vi "UHR-Fleezers Control (host) - 12.6.vi"() -> ()   [LabVIEW 2012] (continued)
      event "Move Cap. 2 (ADig Top)": Value Change {
        n240 = event-data() -> ()  [unwired: 1 in, 5 out]
        n241 = local write "Move Cap. 2 (ADig Top)"(FALSE ("Move Cap. 2 (ADig Left)")) -> ()
        n242 = flat-sequence {
          tunnel: w445 -> [w448]
          tunnel: w446 -> [w449]
          tunnel: [w449] -> w443
          tunnel: [w448] -> w442
          tunnel: w443 -> [w452]
          tunnel: w442 -> [w451]
          frame #0 {
            n243 = property on="Sample Channel\nFlow" class="Bool (strict)"("Val(Sgnl)"="Cap 2 Samp Flow ON") -> ()  [unwired: 2 in, 2 out]
          }
          frame #1 {
            w450 = FALSE ("Value (Signaling)")
            n244 = local read "Saved Stage Positions"() -> (w462:dbl[][])
            n245 = local write "Stage Moving"(TRUE ("Stage Moving")) -> ()
            n246 = Array Subset(array=w462, index (row)=1 ("index"), length (row)=1 ("length"), index (col)=1 ("index"), length (col)=3 ("length")) -> (w459:dbl[][])
            n247 = Reshape Array(w459, 3 ("dimension size")) -> (w457:dbl[])
            n248 = property on="Trap 1 (ON/OFF)" class="Bool (strict)"("Val(Sgnl)"=w450) -> ()  [unwired: 2 in, 2 out]
            n249 = property on="Trap 1 (ON/OFF)" class="Bool (strict)"("Val(Sgnl)"=w450) -> ()  [unwired: 2 in, 2 out]
            n250 = Array To Cluster(array=w457) -> (cluster=w456:cluster{"[0]":dbl, "[1]":dbl, "[2]":dbl})
            n251 = call "Set Stage Position.vi"("Position"=w456, "error in"=w451, "VISA resource name in"=w452) -> ("error out"=w455:errorcluster)  [unwired: 2 out]
            n252 = local write "Stage Control Serial Error"(w455) -> ()
          }
          frame #2 {
            n253 = local write "Stage Moving"(FALSE ("Stage Moving")) -> ()
            n254 = call <vilib>:"Beep.vi"() -> ()  [unwired: 3 in, 9 out]
            n255 = case shown="True" "Cap 2 Flow ON" {
              frame False {
              }
              frame True {
                n256 = property on="Inject Pump 3" class="Bool (strict)"("Val(Sgnl)"=TRUE ("Value (Signaling)")) -> ()  [unwired: 2 in, 2 out]
              }
            }
          }
          frame #3 {
            n257 = property on="Sample Channel\nFlow" class="Bool (strict)"("Val(Sgnl)"=FALSE ("Value (Signaling)")) -> ()  [unwired: 2 in, 2 out]
            n258 = case shown="False" "Cap. 2 BD T1?\n(ADig T1, DNA T2)" {
              tunnel: "Cap 2 T ON" -> [w471 w472]
              frame False {
                n259 = property on="Trap 2 (ON/OFF)" class="Bool (strict)"("Val(Sgnl)"=w471) -> ()  [unwired: 2 in, 2 out]
              }
              frame True {
                n260 = property on="Trap 1 (ON/OFF)" class="Bool (strict)"("Val(Sgnl)"=w472) -> ()  [unwired: 2 in, 2 out]
              }
            }
            n261 = property on="Got ADig bead" class="Bool"("Key Focus"=TRUE) -> ()  [unwired: 2 in, 2 out]
          }
        }
      }
      event "Initialize Blue Laser": Value Change {
        n262 = event-data() -> ()  [unwired: 1 in, 5 out]
        n263 = flat-sequence {
          tunnel: w473 -> [w492]
          frame #0 {
            n264 = Concatenate Strings("slmp ", "Blue Laser\nModulation\nPower (mW)") -> (w491:string)
            n265 = call "serial write macro.vi"("String"=w491, "Delay (ms)"="Delay (ms)", "VISA resource name"=w492) -> ("read buffer"=w480:string, "error out"=w481:errorcluster, "VISA resource name out"=w488:refnum<visa-resource-name>)
            n266 = local write "read blue buffer"(w480) -> ()
            n267 = local write "Blue Error Out"(w481) -> ()
            n268 = call "serial write macro.vi"("String"="sdmes 1", "Delay (ms)"="Delay (ms)", "VISA resource name"=w488) -> ("read buffer"=w478:string, "error out"=w479:errorcluster, "VISA resource name out"=w486:refnum<visa-resource-name>)
            n269 = local write "Blue Error Out"(w479) -> ()
            n270 = local write "read blue buffer"(w478) -> ()
            n271 = call "serial write macro.vi"("String"="sames 1", "Delay (ms)"="Delay (ms)", "VISA resource name"=w486) -> ("read buffer"=w475:string, "error out"=w477:errorcluster, "VISA resource name out"=w483:refnum<visa-resource-name>)
            n272 = local write "read blue buffer"(w475) -> ()
            n273 = local write "Blue Error Out"(w477) -> ()
            n274 = call "serial write macro.vi"("String"="l1", "Delay (ms)"="Delay (ms)", "VISA resource name"=w483) -> ("read buffer"=w474:string, "error out"=w476:errorcluster)  [unwired: 1 out]
            n275 = local write "read blue buffer"(w474) -> ()
            n276 = local write "Blue Error Out"(w476) -> ()
          }
          frame #1 {
            n277 = local write "Initialize Blue Laser"(FALSE ("Initialize")) -> ()
          }
        }
      }
      event "Blue Laser Modluation Mode": Value Change {
        # "Changes the type of modulation for the blue laser"
        n278 = event-data() -> ()  [unwired: 1 in, 5 out]
        n279 = case shown="\"Constant Power\"" "Blue Laser Modluation Mode" {
          tunnel: ["sdmes 1" w510 "sdmes 1" "sdmes 0"] -> w495
          tunnel: ["sames 1" "cp" "sames 0" "sames 1"] -> w494
          frame "Digital + Analog", Default {
          }
          frame "Constant Power" {
            n280 = local read "Blue Laser\nModulation\nPower (mW)"() -> (w513:string)
            n281 = Decimal String To Number(string=w513) -> (number=w509:i32)  [unwired: 2 in, 1 out]
            n282 = Divide(x=w509, y=1000) -> (x/y=w507:dbl)
            n283 = Number To Fractional String(number=w507) -> (F-format string=w508:string)  [unwired: 3 in]
            n284 = Concatenate Strings("p ", w508) -> (w510:string)
          }
          frame "Digital Only" {
          }
          frame "Analog Only" {
          }
        }
        n285 = local read "Delay (ms)"() -> (w504:i32)
        n286 = call "serial write macro.vi"("String"=w495, "Delay (ms)"=w504, "VISA resource name"=w501) -> ("read buffer"=w502:string, "error out"=w503:errorcluster, "VISA resource name out"=w496:refnum<visa-resource-name>)
        n287 = local write "read blue buffer"(w502) -> ()
        n288 = local write "Blue Error Out"(w503) -> ()
        n289 = local read "Delay (ms)"() -> (w499:i32)
        n290 = call "serial write macro.vi"("String"=w494, "Delay (ms)"=w499, "VISA resource name"=w496) -> ("read buffer"=w497:string, "error out"=w498:errorcluster)  [unwired: 1 out]
        n291 = local write "Blue Error Out"(w498) -> ()
        n292 = local write "read blue buffer"(w497) -> ()
      }
      event "Blue Laser\nModulation\nPower (mW)": Value Change {
        n293 = event-data() -> ()  [unwired: 1 in, 5 out]
        n294 = local read "Blue Laser\nModulation\nPower (mW)"() -> (w520:string)
        n295 = local read "Blue Laser Modluation Mode"() -> (w521:string)
        n296 = case shown="\"Constant Power\"" w521 {
          tunnel: w520 -> [w527 w534]
          tunnel: [w526 w533] -> w519
          frame "Constant Power" {
            # "Different command to change constant power instead of modulation power"
            n297 = Decimal String To Number(string=w527) -> (offset past number=w532:i32)  [unwired: 2 in, 1 out]
            n298 = Divide(x=w532, y=1000) -> (x/y=w530:dbl)
            n299 = Number To Fractional String(number=w530) -> (F-format string=w528:string)  [unwired: 3 in]
            n300 = Concatenate Strings("p ", w528) -> (w526:string)
          }
          frame Default {
            n301 = Concatenate Strings("slmp ", w534) -> (w533:string)
          }
        }
        n302 = local read "Delay (ms)"() -> (w524:i32)
        n303 = call "serial write macro.vi"("String"=w519, "Delay (ms)"=w524, "VISA resource name"=w525) -> ("read buffer"=w523:string, "error out"=w522:errorcluster)  [unwired: 1 out]
        n304 = local write "Blue Error Out"(w522) -> ()
        n305 = local write "read blue buffer"(w523) -> ()
      }
      event "Send string\nto Blue Laser": Value Change {
        n306 = event-data() -> ()  [unwired: 1 in, 5 out]
        n307 = flat-sequence {
          tunnel: w536 -> [w541]
          frame #0 {
            n308 = local read "Delay (ms)"() -> (w538:i32)
            n309 = call "serial write macro.vi"("String"="command string", "Delay (ms)"=w538, "VISA resource name"=w541) -> ("read buffer"=w539:string, "error out"=→"Blue Error Out":errorcluster)  [unwired: 1 out]
            "read blue buffer" <- w539
            n310 = String Length(string=w539) -> (length=→"length":i32)
            "command string sent" <- "command string"
          }
          frame #1 {
            n311 = local write "Send string\nto Blue Laser"(FALSE ("Send string")) -> ()
          }
        }
      }
      event "Read Harvard": Value Change {
        n312 = event-data() -> ()  [unwired: 1 in, 5 out]
        n313 = Concatenate Strings("write buffer", "\r") -> (w548:string)
        n314 = VISA Write(VISA resource name=w546, write buffer=w548, error in (no error)=w545) -> (VISA resource name out=w557:refnum<visa-resource-name>, error out=w556:errorcluster)  [unwired: 1 out]
        n315 = stacked-sequence {
          tunnel: [w560] -> w555
          tunnel: w557 -> [w560]
          tunnel: w556 -> [w559]
          tunnel: [w559] -> w550
          frame #0 {
            n316 = Wait (ms)(milliseconds to wait=50) -> ()  [unwired: 1 out]
          }
        }
        n317 = property class="Instr"(reference=w555, error in=w550) -> (reference out=w554:refnum<visa-resource-name>, error out=w552:errorcluster, "Serial Settings:Number of Bytes at Serial Port"=w553:u32)
        "Serial Settings:Number of Bytes at Serial Port" <- w553
        n318 = VISA Read(VISA resource name=w554, byte count=w553, error in (no error)=w552) -> (read buffer=w551:string)  [unwired: 3 out]
        "read buffer" <- w551
        n319 = Fract/Exp String To Number(string=w551) -> ()  [unwired: 5 out]
      }
      event "+z", "-z": Value Change {
        n320 = event-data() -> ()  [unwired: 1 in, 5 out]
        n321 = flat-sequence {
          tunnel: w561 -> [w583]
          tunnel: w562 -> [w563]
          frame #0 {
            n322 = call "Read Stage Position.vi"("error in"=w583, "VISA resource name in"=w563) -> ("Current Position"=w568:cluster{dbl, dbl, dbl}, "error out"=w581:errorcluster, "VISA resource name out"=w582:refnum<visa-resource-name>)  [unwired: 1 out]
            n323 = local read "Saved Stage Positions"() -> (w592:dbl[][])
            n324 = Divide(x="z nudge increment (um)", y=1000.0) -> (x/y=w580:dbl)
            n325 = Boolean To (0,1)(Boolean="+z") -> (0, 1=w572:i16)
            n326 = Boolean To (0,1)(Boolean="-z") -> (0, 1=w573:i16)
            n327 = Array Subset(array=w592, index (row)=1 ("index"), length (row)=1 ("length"), index (col)=1 ("index"), length (col)=3 ("length")) -> (w589:dbl[][])
            n328 = Multiply(x=w572, y=w580) -> (x*y=w576:dbl)
            n329 = Multiply(x=w573, y=w580) -> (x*y=w574:dbl)
            n330 = Unbundle(w568) -> (w566:dbl, w565:dbl, w569:dbl)
            n331 = Negate(x=w574) -> (-x=w575:dbl)
            n332 = Reshape Array(w589, 3 ("dimension size")) -> (w587:dbl[])
            n333 = Add(x=w576, y=w575) -> (x+y=w577:dbl)
            n334 = Array To Cluster(array=w587) -> ()  [unwired: 1 out]
            n335 = Add(x=w577, y=w569) -> (x+y=w567:dbl)
            n336 = Bundle(cluster=w568, w566, w565, w567) -> (w564:cluster{dbl, dbl, dbl})
            n337 = call "Set Stage Position.vi"("Position"=w564, "error in"=w581, "VISA resource name in"=w582) -> ("error out"=w586:errorcluster)  [unwired: 2 out]
            n338 = local write "Stage Moving"(TRUE ("Stage Moving")) -> ()
            n339 = local write "Stage Control Serial Error"(w586) -> ()
          }
          frame #1 {
            n340 = local write "Stage Moving"(FALSE ("Stage Moving")) -> ()
            n341 = call <vilib>:"Beep.vi"() -> ()  [unwired: 3 in, 9 out]
          }
        }
      }
      event "Cal/Data Acq. Spot": Value Change {
        n342 = event-data() -> ()  [unwired: 1 in, 5 out]
        n343 = flat-sequence {
          tunnel: w601 -> [w605]
          tunnel: w602 -> [w606]
          tunnel: [w606] -> w598
          tunnel: [w605] -> w597
          tunnel: w598 -> [w611]
          tunnel: w597 -> [w610]
          tunnel: ["Cal @ (MHz)"] -> w595
          tunnel: [w615] -> w599
          tunnel: w595 -> [w615]
          tunnel: w599 -> [w624]
          tunnel: ["W/ Offset 1"] -> w596
          tunnel: w599 -> [w645]
          tunnel: w596 -> [w643]
          frame #0 {
            n344 = property on="Sample Channel\nFlow" class="Bool (strict)"("Val(Sgnl)"="Daq spot flow on") -> ()  [unwired: 2 in, 2 out]
            n345 = Wait (ms)(milliseconds to wait=u32 250) -> ()  [unwired: 1 out]
          }
          frame #1 {
            n346 = local read "Saved Stage Positions"() -> (w608:dbl[][])
            n347 = property on="Trap Delta (MHz)" class="DigNum (strict)"("Val(Sgnl)"="Cal @ (MHz)") -> ()  [unwired: 2 in, 2 out]
            n348 = local write "Stage Moving"(TRUE ("Stage Moving")) -> ()
            n349 = call "move to saved stage position.vi"("error in"=w610, "Stage VISA resource name in"=w611, "Position"="Cal Stage Position", "Saved Stage Positions"=w608) -> ("error out"=w609:errorcluster)  [unwired: 1 out]
            n350 = local write "Stage Control Serial Error"(w609) -> ()
          }
          frame #2 {
            n351 = local write "Stage Moving"(FALSE ("Stage Moving")) -> ()
            n352 = property on="Sample Channel\nFlow" class="Bool (strict)"("Val(Sgnl)"="Flow ON during cal?") -> ()  [unwired: 2 in, 2 out]
            n353 = call <vilib>:"Beep.vi"() -> ()  [unwired: 3 in, 9 out]
          }
          frame #3 {
            n354 = Wait (ms)(milliseconds to wait=u32 1000) -> ()  [unwired: 1 out]
          }
          frame #4 {
            n355 = property on="Save Calibration" class="Bool (strict)"("Val(Sgnl)"=TRUE ("Value (Signaling)")) -> ()  [unwired: 2 in, 2 out]
          }
          frame #5 {
            n356 = Wait (ms)(milliseconds to wait=u32 2000) -> ()  [unwired: 1 out]
          }
          frame #6 {
            # "Check to see if \nsaving done"
            n357 = while {
              stop <- w620 stop-if-true
              n358 = local read "Saving..."() -> (w621:bool)
              n359 = Wait (ms)(milliseconds to wait=u32 100) -> ()  [unwired: 1 out]
              n360 = Not(x=w621) -> (.not. x?=w620:bool)
            }
          }
          frame #7 {
            n361 = case shown="True" "W/ Offset 1" {
              tunnel: w624 -> [_ w625]
              frame False {
              }
              frame True {
                n362 = stacked-sequence {
                  tunnel: w625 -> [_ _ _ _ _ _ _ w642]
                  frame #0 {
                    n363 = property on="Trap Delta (MHz)" class="DigNum (strict)"("Val(Sgnl)"="Offset 1 Start (MHz)") -> ()  [unwired: 2 in, 2 out]
                    n364 = Replace Array Subset(array=u32[] [0] ("Index Values"), new element="Offset 1 Set", index=0) -> (w626:u32[])
                    n365 = property on="Saved AOD Raster Scan Parameter Sets" class="Arr (strict)"("Index Values"=w626) -> ()  [unwired: 2 in, 2 out]
                  }
                  frame #1 {
                    n366 = Wait (ms)(milliseconds to wait=u32 200) -> ()  [unwired: 1 out]
                  }
                  frame #2 {
                    n367 = property on="Load parameters" class="Bool (strict)"("Val(Sgnl)"=TRUE ("Value (Signaling)")) -> ()  [unwired: 2 in, 2 out]
                  }
                  frame #3 {
                    n368 = Wait (ms)(milliseconds to wait=u32 200) -> ()  [unwired: 1 out]
                  }
                  frame #4 {
                    n369 = property on="Trap Raster Scan" class="Bool (strict)"("Val(Sgnl)"=TRUE ("Value (Signaling)")) -> ()  [unwired: 2 in, 2 out]
                  }
                  frame #5 {
                    n370 = Wait (ms)(milliseconds to wait=u32 2000) -> ()  [unwired: 1 out]
                  }
                  frame #6 {
                    n371 = while {
                      stop <- w639 stop-if-true
                      n372 = local read "Raster Scanning..."() -> (w641:bool)
                      n373 = local read "Saving..."() -> (w637:bool)
                      n374 = Wait (ms)(milliseconds to wait=u32 100) -> ()  [unwired: 1 out]
                      n375 = Not(x=w637) -> (.not. x?=w636:bool)
                      n376 = Not(x=w641) -> (.not. x?=w638:bool)
                      n377 = And(x=w638, y=w636) -> (x .and. y?=w639:bool)
                    }
                  }
                  frame #7 {
                    n378 = property on="Trap Delta (MHz)" class="DigNum (strict)"("Val(Sgnl)"=w642) -> ()  [unwired: 2 in, 2 out]
                  }
                }
              }
            }
          }
          frame #8 {
            n379 = local read "Save ave N"() -> (w644:dbl)
            n380 = case shown="False" "W/ Offset 2" {
              tunnel: w645 -> [_ w652]
              tunnel: w644 -> [_ w651]
              tunnel: w643 -> [w647 _]
              frame False {
                n381 = case shown="False" w647 {
                  frame False {
                    n382 = Multiply(x="Cal read wait (s)", y=u32 1000 ("milliseconds to wait")) -> (x*y=w649:u32)
                    n383 = Wait (ms)(milliseconds to wait=w649) -> ()  [unwired: 1 out]
                  }
                  frame True {
                  }
                }
              }
              frame True {
                n384 = stacked-sequence {
                  tunnel: w652 -> [_ _ _ _ _ _ _ _ _ w673 _ _]
                  tunnel: w651 -> [_ _ _ _ _ _ _ _ _ w671 _ _]
                  frame #0 {
                    n385 = property on="Save ave N" class="DigNum (strict)"("Val(Sgnl)"=1.0 ("Value (Signaling)")) -> ()  [unwired: 2 in, 2 out]
                  }
                  frame #1 {
                    n386 = Wait (ms)(milliseconds to wait=u32 500) -> ()  [unwired: 1 out]
                  }
                  frame #2 {
                    n387 = property on="Trap Delta (MHz)" class="DigNum (strict)"("Val(Sgnl)"="Offset 2 Start (MHz)") -> ()  [unwired: 2 in, 2 out]
                    n388 = Replace Array Subset(array=u32[] [0] ("Index Values"), new element="Offset 2 Set", index=0) -> (w657:u32[])
                    n389 = property on="Saved AOD Raster Scan Parameter Sets" class="Arr (strict)"("Index Values"=w657) -> ()  [unwired: 2 in, 2 out]
                  }
                  frame #3 {
                    n390 = Wait (ms)(milliseconds to wait=u32 500) -> ()  [unwired: 1 out]
                  }
                  frame #4 {
                    n391 = property on="Load parameters" class="Bool (strict)"("Val(Sgnl)"=TRUE ("Value (Signaling)")) -> ()  [unwired: 2 in, 2 out]
                  }
                  frame #5 {
                    n392 = Wait (ms)(milliseconds to wait=u32 500) -> ()  [unwired: 1 out]
                  }
                  frame #6 {
                    n393 = property on="Trap Raster Scan" class="Bool (strict)"("Val(Sgnl)"=TRUE ("Value (Signaling)")) -> ()  [unwired: 2 in, 2 out]
                  }
                  frame #7 {
                    n394 = Wait (ms)(milliseconds to wait=u32 2000) -> ()  [unwired: 1 out]
                  }
                  frame #8 {
                    n395 = while {
                      stop <- w666 stop-if-true
                      n396 = local read "Raster Scanning..."() -> (w669:bool)
                      n397 = local read "Saving..."() -> (w667:bool)
                      n398 = Wait (ms)(milliseconds to wait=u32 100) -> ()  [unwired: 1 out]
                      n399 = Not(x=w667) -> (.not. x?=w665:bool)
                      n400 = Not(x=w669) -> (.not. x?=w668:bool)
                      n401 = And(x=w668, y=w665) -> (x .and. y?=w666:bool)
                    }
                  }
                  frame #9 {
                    n402 = property on="Trap Delta (MHz)" class="DigNum (strict)"("Val(Sgnl)"=w673) -> ()  [unwired: 2 in, 2 out]
                    n403 = property on="Saved AOD Raster Scan Parameter Sets" class="Arr (strict)"("Index Values"=u32[] [0]) -> ()  [unwired: 2 in, 2 out]
                    n404 = property on="Save ave N" class="DigNum (strict)"("Val(Sgnl)"=w671) -> ()  [unwired: 2 in, 2 out]
                  }
                  frame #10 {
                    n405 = Wait (ms)(milliseconds to wait=u32 500) -> ()  [unwired: 1 out]
                  }
                  frame #11 {
                    n406 = property on="Load parameters" class="Bool (strict)"("Val(Sgnl)"=TRUE ("Value (Signaling)")) -> ()  [unwired: 2 in, 2 out]
                  }
                }
              }
            }
          }
          frame #9 {
            n407 = property on="Read Cal" class="Bool (strict)"("Val(Sgnl)"=TRUE ("Value (Signaling)")) -> ()  [unwired: 2 in, 2 out]
          }
          frame #10 {
            n408 = Wait (ms)(milliseconds to wait=u32 1000) -> ()  [unwired: 1 out]
          }
          frame #11 {
            n409 = property on="Fish for Tether" class="Bool (strict)"("Val(Sgnl)"=TRUE ("Value (Signaling)")) -> ()  [unwired: 2 in, 2 out]
          }
        }
        n410 = local write "Cal/Data Acq. Spot"(FALSE ("Cal/Data Acq. Spot")) -> ()
      }
      event "Dump Beads": Value Change {
        n411 = event-data() -> ()  [unwired: 1 in, 5 out]
        n412 = flat-sequence {
          tunnel: ["Dump spot flow on?"] -> w679
          tunnel: [w690] -> w680
          tunnel: w679 -> [w690]
          tunnel: w683 -> [w695]
          tunnel: w682 -> [w694]
          tunnel: [w692] -> w681
          tunnel: w680 -> [w692]
          tunnel: w681 -> [w705]
          frame #0 {
            w684 = FALSE ("Value (Signaling)")
            n413 = local read "Saving..."() -> (w686:bool)
            n414 = local write "Dump Beads"(FALSE ("Dump Beads")) -> ()
            n415 = property on="Inject Pump 3" class="Bool (strict)"("Val(Sgnl)"=w684) -> ()  [unwired: 2 in, 2 out]
            n416 = property on="Inject Pump 1" class="Bool (strict)"("Val(Sgnl)"=w684) -> ()  [unwired: 2 in, 2 out]
            n417 = local write "Stop Saving"(w686) -> ()
          }
          frame #1 {
            w687 = FALSE ("Fl. Triggered...")
            n418 = case shown="True" "Dump spot flow on?" {
              frame False {
              }
              frame True {
                n419 = property on="Sample Channel\nFlow" class="Bool (strict)"("Val(Sgnl)"=TRUE ("Stage Moving")) -> ()  [unwired: 2 in, 2 out]
              }
            }
            n420 = local write "Fl. Triggered..."(w687) -> ()
            n421 = local write "Tether"(w687) -> ()
            n422 = property on="Green Laser ON" class="Bool (strict)"("Val(Sgnl)"=w687) -> ()  [unwired: 2 in, 2 out]
            n423 = property on="Trap Pos. FB ON" class="Bool (strict)"("Val(Sgnl)"=w687) -> ()  [unwired: 2 in, 2 out]
            n424 = property on="Trap Trig. Fl." class="Bool (strict)"("Val(Sgnl)"=w687) -> ()  [unwired: 2 in, 2 out]
            n425 = property on="Fl. Triggered..." class="Bool (strict)"("Val(Sgnl)"=w687) -> ()  [unwired: 2 in, 2 out]
            n426 = property on="Dip for Protein" class="Bool (strict)"("Val(Sgnl)"=w687) -> ()  [unwired: 2 in, 2 out]
            n427 = property on="Pause dwell" class="Bool (strict)"("Val(Sgnl)"=w687) -> ()  [unwired: 2 in, 2 out]
          }
          frame #2 {
            n428 = property on="Trap Pos. FB Offset Factor" class="DigNum (strict)"("Val(Sgnl)"=i64 0 ("Value (Signaling)")) -> ()  [unwired: 2 in, 2 out]
          }
          frame #3 {
            n429 = local read "Saved Stage Positions"() -> (w696:dbl[][])
            n430 = local write "Stage Moving"(TRUE ("Stage Moving")) -> ()
            n431 = Array Subset(array=w696, index (row)=3 ("index"), length (row)=1 ("length"), index (col)=1 ("index"), length (col)=3 ("length")) -> (w701:dbl[][])
            n432 = Reshape Array(w701, 3 ("dimension size")) -> (w699:dbl[])
            n433 = Array To Cluster(array=w699) -> (cluster=w698:cluster{"[0]":dbl, "[1]":dbl, "[2]":dbl})
            n434 = call "Set Stage Position.vi"("Position"=w698, "error in"=w694, "VISA resource name in"=w695) -> ()  [unwired: 3 out]
          }
          frame #4 {
            w706 = FALSE ("Value (Signaling)")
            n435 = case shown="True" w705 {
              frame False {
              }
              frame True {
                n436 = property on="Sample Channel\nFlow" class="Bool (strict)"("Val(Sgnl)"=FALSE ("Stage Moving")) -> ()  [unwired: 2 in, 2 out]
              }
            }
            n437 = property on="Trap 1 (ON/OFF)" class="Bool (strict)"("Val(Sgnl)"=w706) -> ()  [unwired: 2 in, 2 out]
            n438 = property on="Trap 2 (ON/OFF)" class="Bool (strict)"("Val(Sgnl)"=w706) -> ()  [unwired: 2 in, 2 out]
            n439 = call <vilib>:"Beep.vi"() -> ()  [unwired: 3 in, 9 out]
          }
          frame #5 {
            n440 = property on="Move Cap. 2 (ADig Top)" class="Bool (strict)"("Val(Sgnl)"=TRUE ("Value (Signaling)")) -> ()  [unwired: 2 in, 2 out]
            n441 = property on="Tab Control" class="TabCtl (strict)"("Val(Sgnl)"=T26."Status" ("Value (Signaling)")) -> ()  [unwired: 2 in, 2 out]
          }
        }
      }
      event "Dip for Protein": Value Change {
        n442 = event-data() -> ()  [unwired: 1 in, 5 out]
        n443 = case shown="True" "Dip for Protein" {
          tunnel: w712 -> [_ w714]
          tunnel: w711 -> [_ w713]
          frame False {
          }
          frame True {
            n444 = while {
              tunnel: w714 -> [w725]
              tunnel: w713 -> [w724]
              i -> [w719]
              stop <- w721 stop-if-true
              n445 = Increment(x=w719) -> (x+1=→"Dip #":i32)
              n446 = flat-sequence {
                tunnel: w724 -> [w736]
                tunnel: w725 -> [w737]
                tunnel: [w737] -> w729
                tunnel: [w736] -> w728
                tunnel: [w730] -> w715
                tunnel: [w742] -> w723
                tunnel: [w743] -> w722
                tunnel: w729 -> [w744]
                tunnel: w728 -> [w745]
                tunnel: [w740] -> w716
                tunnel: w715 -> [w740]
                tunnel: [w753] -> w727
                tunnel: w723 -> [w753]
                tunnel: [w752] -> w726
                tunnel: w722 -> [w752]
                tunnel: [w749] -> w720
                tunnel: [w748] -> w717
                tunnel: w716 -> [w748]
                tunnel: w726 -> [w773]
                tunnel: w727 -> [w774]
                tunnel: w720 -> [w775]
                tunnel: w717 -> [w772]
                tunnel: [w831] -> w721
                frame #0 {
                  n447 = local read "Trap Pos. FB ON"() -> (w730:bool)
                  n448 = Compound Arithmetic op=AND("Flow ON\nduring dip?", "FB OFF when \nflow ON", w730) -> (w731:bool)
                  n449 = case shown="True" "Move trap \nbefore dip move?" {
                    frame False {
                    }
                    frame True {
                      n450 = property on="Trap Delta (MHz)" class="DigNum (strict)"("Val(Sgnl)"="Dipping Delta (MHz)") -> ()  [unwired: 2 in, 2 out]
                    }
                  }
                  n451 = property on="Green Laser ON" class="Bool (strict)"("Val(Sgnl)"="Green ON\nbefore dip?") -> ()  [unwired: 2 in, 2 out]
                  n452 = property on="Sample Channel\nFlow" class="Bool (strict)"("Val(Sgnl)"="Flow ON\nduring dip?") -> ()  [unwired: 2 in, 2 out]
                  n453 = case shown="True" w731 {
                    frame False {
                    }
                    frame True {
                      n454 = property on="Trap Pos. FB ON" class="Bool (strict)"("Val(Sgnl)"=FALSE ("Value (Signaling)")) -> ()  [unwired: 2 in, 2 out]
                    }
                  }
                }
                frame #1 {
                  n455 = local read "Saved Stage Positions"() -> (w747:dbl[][])
                  n456 = local write "Cancel dwell"(FALSE ("Cancel dwell")) -> ()
                  n457 = call "move to saved stage position.vi"("error in"=w745, "Stage VISA resource name in"=w744, "Position"="Dip Stage \nPosition", "Saved Stage Positions"=w747) -> ("VISA resource name out"=w742:refnum<visa-resource-name>, "error out"=w743:errorcluster)
                }
                frame #2 {
                  n458 = node-c288() -> (w751:T23)  [unwired: 4 in]
                  n459 = timed-loop {
                    timing: w751 -> [_]
                    timing-out: [_] -> w750
                    tunnel: [w757] -> w749
                    i -> [w754]
                    stop <- w758 stop-if-true
                    n460 = node-c288() -> ()  [unwired: 1 in, 1 out]
                    n461 = Greater Or Equal?(x=w754, y="Dip Duration (s)") -> (x >= y?=w766:bool)
                    n462 = local read "Dip for Protein"() -> (w759:bool)
                    n463 = local read "Dump Beads"() -> (w756:bool)
                    n464 = local read "Cancel dwell"() -> (w765:bool)
                    n465 = local read "Pause dwell"() -> (w762:bool)
                    n466 = Not(x=w759) -> (.not. x?=w764:bool)
                    n467 = Compound Arithmetic op=OR(w765, w766, w764) -> (w763:bool)
                    n468 = Select(t=FALSE, s=w762, f=w763) -> (s? t:f=w760:bool)
                    n469 = Not(x=w756) -> (.not. x?=w755:bool)
                    n470 = node-c288() -> ()  [unwired: 1 in, 1 out]
                    n471 = And(x=w759, y=w755) -> (x .and. y?=w757:bool)
                    n472 = Or(x=w760, y=w756) -> (x .or. y?=w758:bool)
                    "Dip Time (s)" <- w754
                  }
                  n473 = node-c288(w750) -> ()  [unwired: 1 out]
                }
                frame #3 {
                  n474 = case shown="True" w775 {
                    tunnel: w774 -> [_ w780]
                    tunnel: w773 -> [_ w779]
                    tunnel: w772 -> [_ w776]
                    frame False {
                    }
                    frame True {
                      n475 = flat-sequence {
                        tunnel: w779 -> [w784]
                        tunnel: w780 -> [w785]
                        tunnel: [w785] -> w778
                        tunnel: [w784] -> w777
                        tunnel: w776 -> [w781]
                        tunnel: w778 -> [w795]
                        tunnel: w777 -> [w794]
                        tunnel: w776 -> [w803]
                        frame #0 {
                          n476 = local read "Sample Channel\nFlow"() -> (w783:bool)
                          n477 = case shown="True" w783 {
                            tunnel: "Flow ON \nduring return\nfrom dip?" -> [w786 w789]
                            tunnel: w781 -> [_ w788]
                            frame False {
                              n478 = case shown="True" w786 {
                                frame False {
                                }
                                frame True {
                                n479 = property on="Sample Channel\nFlow" class="Bool (strict)"("Val(Sgnl)"=TRUE ("Value (Signaling)")) -> ()  [unwired: 2 in, 2 out]
                                }
                              }
                            }
                            frame True {
                              n480 = case shown="False" w789 {
                                tunnel: w788 -> [w790 _]
                                frame False {
                                n481 = property on="Trap Pos. FB ON" class="Bool (strict)"("Val(Sgnl)"=w790) -> ()  [unwired: 2 in, 2 out]
                                n482 = property on="Sample Channel\nFlow" class="Bool (strict)"("Val(Sgnl)"=FALSE ("Value (Signaling)")) -> ()  [unwired: 2 in, 2 out]
                                }
                                frame True {
                                }
                              }
                            }
                          }
                        }
                        frame #1 {
                          # "For turning on green laser before stage reaches lower spot"
                          n483 = case shown="True" "Green ON\nafter start\nreturn?" {
                            frame False {
                            }
                            frame True {
                              n484 = flat-sequence {
                                frame #0 {
                                n485 = Multiply(x="Green delay after \nstart return (s)", y=1000.0) -> (x*y=w800:dbl)
                                n486 = Wait (ms)(milliseconds to wait=w800) -> ()  [unwired: 1 out]
                                }
                                frame #1 {
                                n487 = property on="Green Laser ON" class="Bool (strict)"("Val(Sgnl)"=TRUE ("Value (Signaling)")) -> ()  [unwired: 2 in, 2 out]
                                }
                              }
                            }
                          }
                          n488 = local read "Saved Stage Positions"() -> (w798:dbl[][])
                          n489 = local write "Cancel dwell"(FALSE ("Cancel dwell")) -> ()
                          n490 = call "move to saved stage position.vi"("error in"=w794, "Stage VISA resource name in"=w795, "Position"="Return Stage \nPosition", "Saved Stage Positions"=w798) -> ("error out"=w796:errorcluster)  [unwired: 1 out]
                          n491 = local write "Stage Control Serial Error"(w796) -> ()
                        }
                        frame #2 {
                          n492 = property on="Trap Pos. FB ON" class="Bool (strict)"("Val(Sgnl)"=w803) -> ()  [unwired: 2 in, 2 out]
                          n493 = case shown="True" "Green ON \nafter return?" {
                            frame False {
                            }
                            frame True {
                              n494 = property on="Green Laser ON" class="Bool (strict)"("Val(Sgnl)"=TRUE ("Value (Signaling)")) -> ()  [unwired: 2 in, 2 out]
                            }
                          }
                          n495 = case shown="True" "Move trap after return?" {
                            frame False {
                            }
                            frame True {
                              n496 = property on="Trap Delta (MHz)" class="DigNum (strict)"("Val(Sgnl)"="Dip Trap Delta 2 (MHz)") -> ()  [unwired: 2 in, 2 out]
                            }
                          }
                          n497 = case shown="True" "Save data after return?" {
                            frame False {
                            }
                            frame True {
                              n498 = property on="Start Saving" class="Bool (strict)"("Val(Sgnl)"=TRUE ("Value (Signaling)")) -> ()  [unwired: 2 in, 2 out]
                            }
                          }
                          n499 = property on="Sample Channel\nFlow" class="Bool (strict)"("Val(Sgnl)"="Flow ON\nduring daq?") -> ()  [unwired: 2 in, 2 out]
                        }
                        frame #3 {
                          n500 = node-c288() -> (w812:T23)  [unwired: 4 in]
                          n501 = timed-loop {
                            timing: w812 -> [_]
                            timing-out: [_] -> w811
                            i -> [w813]
                            stop <- w815 stop-if-true
                            n502 = node-c288() -> ()  [unwired: 1 in, 1 out]
                            n503 = local read "Dump Beads"() -> (w814:bool)
                            n504 = Greater Or Equal?(x=w813, y="Dwell Duration (s)") -> (x >= y?=w820:bool)
                            n505 = local read "Dip for Protein"() -> (w817:bool)
                            n506 = Not(x=w817) -> (.not. x?=w816:bool)
                            n507 = Compound Arithmetic op=OR(w820, "Cancel dwell", w816) -> (w819:bool)
                            n508 = node-c288() -> ()  [unwired: 1 in, 1 out]
                            n509 = Select(t=FALSE, s="Pause dwell", f=w819) -> (s? t:f=w822:bool)
                            n510 = Or(x=w822, y=w814) -> (x .or. y?=w815:bool)
                            "Dwell Time (s)" <- w813
                          }
                          n511 = node-c288(w811) -> ()  [unwired: 1 out]
                        }
                      }
                    }
                  }
                }
                frame #4 {
                  n512 = local read "Dip for Protein"() -> (w832:bool)
                  n513 = local read "Dump Beads"() -> (w829:bool)
                  n514 = local write "Cancel dwell"(FALSE ("Cancel dwell")) -> ()
                  n515 = Not(x=w832) -> (.not. x?=w833:bool)
                  n516 = Not(x="Cont. Repeat Dipping?") -> (.not. x?=w835:bool)
                  n517 = Compound Arithmetic op=OR(w833, w835, w829) -> (w831:bool)
                }
              }
            }
          }
        }
      }
      event "Profile": Value Change {
        n518 = event-data() -> ()  [unwired: 1 in, 5 out]
        n519 = flat-sequence {
          tunnel: w844 -> [w847]
          tunnel: w843 -> [w855]
          tunnel: [w849] -> w842
          tunnel: [w848] -> w841
          tunnel: [w846] -> w839
          tunnel: [w845] -> w836
          tunnel: w842 -> [w862]
          tunnel: w841 -> [w861]
          tunnel: [w859] -> w840
          tunnel: w839 -> [w860]
          tunnel: [w858] -> w838
          tunnel: [w857] -> w837
          tunnel: w836 -> [w857]
          tunnel: w840 -> [w866]
          tunnel: w838 -> [w865]
          tunnel: w837 -> [w864]
          frame #0 {
            n520 = call "Read Stage Position.vi"("error in"=w855, "VISA resource name in"=w847) -> ("Current Position"=w845:cluster{dbl, dbl, dbl}, "error out"=w848:errorcluster, "VISA resource name out"=w846:refnum<visa-resource-name>)  [unwired: 1 out]
            "Current Position" <- w845
            n521 = local write "Stage Control Serial Error"(w848) -> ()
            n522 = Unbundle(w845) -> (w852:dbl, w854:dbl, w850:dbl)
            n523 = Add(x=w854, y="Y change (mm)") -> (x+y=w851:dbl)
            n524 = Bundle(w852, w851, w850) -> (w849:cluster{dbl, dbl, dbl})  [unwired: 1 in]
          }
          frame #1 {
            # "move to new position and start saving"
            n525 = local write "Stage Moving"(TRUE ("Stage Moving")) -> ()
            n526 = local write "Start Saving"(TRUE ("Start Saving")) -> ()
            n527 = call "Set Stage Position.vi"("Position"=w862, "error in"=w861, "VISA resource name in"=w860) -> ("error out"=w858:errorcluster, "VISA resource name out"=w859:refnum<visa-resource-name>)  [unwired: 1 out]
          }
          frame #2 {
            # "go back to start"
            n528 = call "Set Stage Position.vi"("Position"=w864, "error in"=w865, "VISA resource name in"=w866) -> ()  [unwired: 3 out]
          }
          frame #3 {
            # "stop saving"
            n529 = local write "Stop Saving"(TRUE ("Stop Saving")) -> ()
            n530 = local write "Stage Moving"(FALSE ("Stage Moving")) -> ()
          }
        }
      }
      event "Move to Position 1", "Move to Position 2", "Move to Position 3", "Move to Position 4", "Move to Position 5", "Lower Ch. Cap.": Value Change {
        n531 = event-data() -> ()  [unwired: 1 in, 5 out]
        n532 = Or(x="Move to Position 5", y="Lower Ch. Cap.") -> (x .or. y?=w872:bool)
        n533 = Build Array("Move to Position 1", "Move to Position 2", "Move to Position 3", "Move to Position 4", w872) -> (w875:bool[])
        n534 = Boolean Array To Number(Boolean array=w875) -> (number=w874:u32)
        n535 = Logarithm Base 2(1:w874) -> (0:w873:dbl)
        n536 = flat-sequence {
          tunnel: w873 -> [w884]
          tunnel: w870 -> [w882]
          tunnel: w869 -> [w881]
          frame #0 {
            n537 = local read "Saved Stage Positions"() -> (w892:dbl[][])
            n538 = Array Subset(array=w892, index (row)=w884, length (row)=1 ("length"), index (col)=1 ("index"), length (col)=3 ("length")) -> (w889:dbl[][])
            n539 = Reshape Array(w889, 3 ("dimension size")) -> (w887:dbl[])
            n540 = Array To Cluster(array=w887) -> (cluster=w886:cluster{"[0]":dbl, "[1]":dbl, "[2]":dbl})
            n541 = call "Set Stage Position.vi"("Position"=w886, "error in"=w881, "VISA resource name in"=w882) -> ("error out"=w885:errorcluster)  [unwired: 2 out]
            n542 = local write "Stage Moving"(TRUE ("Stage Moving")) -> ()
            n543 = local write "Stage Control Serial Error"(w885) -> ()
          }
          frame #1 {
            n544 = local write "Stage Moving"(FALSE ("Stage Moving")) -> ()
            n545 = call <vilib>:"Beep.vi"() -> ()  [unwired: 3 in, 9 out]
          }
        }
      }
      event "Got ADig bead": Value Change {
        n546 = event-data() -> ()  [unwired: 1 in, 5 out]
        n547 = flat-sequence {
          frame #0 {
            n548 = local read "Cap 1 Samp Flow ON"() -> (w896:bool)
            n549 = case shown="True" w896 {
              frame False {
              }
              frame True {
                n550 = property on="Sample Channel\nFlow" class="Bool (strict)"("Val(Sgnl)"=TRUE ("Value (Signaling)")) -> ()  [unwired: 2 in, 2 out]
              }
            }
          }
          frame #1 {
            n551 = property on="Inject Pump 3" class="Bool (strict)"("Val(Sgnl)"=FALSE ("Value (Signaling)")) -> ()  [unwired: 2 in, 2 out]
          }
          frame #2 {
            n552 = property on="Move Cap. 1 (DNA Bottom)" class="Bool (strict)"("Val(Sgnl)"=TRUE ("Value (Signaling)")) -> ()  [unwired: 2 in, 2 out]
          }
        }
      }
      event "Force FB Data\nScript": Value Change {
        n553 = event-data() -> ()  [unwired: 1 in, 5 out]
        n554 = flat-sequence {
          tunnel: w905 -> [w909]
          tunnel: w906 -> [w910]
          tunnel: [w910] -> w901
          tunnel: [w909] -> w900
          tunnel: w901 -> [w913]
          tunnel: w900 -> [w912]
          tunnel: ["Trap Trig Fl."] -> w902
          tunnel: [w938] -> w903
          tunnel: w902 -> [w938]
          tunnel: [w942] -> w904
          tunnel: w903 -> [w942]
          tunnel: w904 -> [w944]
          frame #0 {
            n555 = property on="Trap Delta (MHz)" class="DigNum (strict)"("Val(Sgnl)"="Trap Delta Before Moving") -> ()  [unwired: 2 in, 2 out]
          }
          frame #1 {
            n556 = local read "Saved Stage Positions"() -> (w915:dbl[][])
            n557 = local write "FB Trap Pos Offset"(0.0 ("FB Trap Pos Offset")) -> ()
            n558 = property on="Trap Pos. FB Offset Factor" class="DigNum (strict)"("Val(Sgnl)"=i64 0 ("Value (Signaling)")) -> ()  [unwired: 2 in, 2 out]
            n559 = local write "Stage Moving"(TRUE ("Stage Moving")) -> ()
            n560 = call "move to saved stage position.vi"("error in"=w912, "Stage VISA resource name in"=w913, "Position"="Stage Position To Establish FB", "Saved Stage Positions"=w915) -> ("error out"=w911:errorcluster)  [unwired: 1 out]
            n561 = local write "Stage Control Serial Error"(w911) -> ()
          }
          frame #2 {
            n562 = call <vilib>:"Beep.vi"() -> ()  [unwired: 3 in, 9 out]
            n563 = Multiply(x="Wait (s)", y=u32 1000 ("milliseconds to wait")) -> (x*y=w922:u32)
            n564 = property on="Trap Delta (MHz)" class="DigNum (strict)"("Val(Sgnl)"="Starting \nTrap Delta (MHz)") -> ()  [unwired: 2 in, 2 out]
            n565 = local write "Stage Moving"(FALSE ("Stage Moving")) -> ()
            n566 = Wait (ms)(milliseconds to wait=w922) -> ()  [unwired: 1 out]
            n567 = property on="Tab Control 2" class="TabCtl (strict)"("Val(Sgnl)"=T6."Feedback on Trap Position" ("Value (Signaling)")) -> ()  [unwired: 2 in, 2 out]
            n568 = property on="Tab Control" class="TabCtl (strict)"("Val(Sgnl)"=T27."Trap Control (RF)" ("Value (Signaling)")) -> ()  [unwired: 2 in, 2 out]
          }
          frame #3 {
            n569 = property on="Set Reading to\nSetpoint" class="Bool (strict)"("Val(Sgnl)"=TRUE ("Value (Signaling)")) -> ()  [unwired: 2 in, 2 out]
            n570 = Wait (ms)(milliseconds to wait=u32 500) -> ()  [unwired: 1 out]
          }
          frame #4 {
            n571 = property on="Trap Pos. FB ON" class="Bool (strict)"("Val(Sgnl)"=TRUE ("Value (Signaling)")) -> ()  [unwired: 2 in, 2 out]
            n572 = Wait (ms)(milliseconds to wait=u32 250) -> ()  [unwired: 1 out]
          }
          frame #5 {
            n573 = case shown="False" "Trap Trig Fl." {
              frame False {
                n574 = case shown="True" "Green ON after FB ON?" {
                  selector: "Green ON after FB ON?" -> [_ w937]
                  frame False {
                  }
                  frame True {
                    n575 = property on="Green Laser ON" class="Bool (strict)"("Val(Sgnl)"=w937) -> ()  [unwired: 2 in, 2 out]
                  }
                }
              }
              frame True {
              }
            }
            n576 = case shown="True" "Remove Action Offset" {
              tunnel: TRUE ("Value (Signaling)") -> [w934 w935]
              frame False {
                n577 = property on="Remove Unwinding Offset" class="Bool (strict)"("Val(Sgnl)"=w934) -> ()  [unwired: 2 in, 2 out]
              }
              frame True {
                n578 = property on="Remove Action Offset" class="Bool (strict)"("Val(Sgnl)"=w935) -> ()  [unwired: 2 in, 2 out]
              }
            }
            n579 = Wait (ms)(milliseconds to wait=u32 250) -> ()  [unwired: 1 out]
          }
          frame #6 {
            n580 = property on="Start Saving" class="Bool (strict)"("Val(Sgnl)"=TRUE ("Value (Signaling)")) -> ()  [unwired: 2 in, 2 out]
            n581 = Wait (ms)(milliseconds to wait=u32 5000) -> ()  [unwired: 1 out]
          }
          frame #7 {
            w941 = TRUE ("Value (Signaling)")
            n582 = property on="Rem fb disp offset" class="Bool (strict)"("Val(Sgnl)"=w941) -> ()  [unwired: 2 in, 2 out]
            n583 = property on="Remove Offset" class="Bool (strict)"("Val(Sgnl)"=w941) -> ()  [unwired: 2 in, 2 out]
            n584 = Wait (ms)(milliseconds to wait=u32 100) -> ()  [unwired: 1 out]
          }
          frame #8 {
            n585 = case shown="True" w944 {
              frame False {
              }
              frame True {
                n586 = local write "Trap Trig. Fl."(TRUE ("Value (Signaling)")) -> ()
              }
            }
          }
          frame #9 {
            n587 = case shown="True" "Start dipping after?" {
              frame False {
              }
              frame True {
                n588 = flat-sequence {
                  frame #0 {
                    n589 = Multiply(x="Delay before dipping (s)", y=1000.0) -> (x*y=w948:dbl)
                    n590 = Wait (ms)(milliseconds to wait=w948) -> ()  [unwired: 1 out]
                  }
                  frame #1 {
                    n591 = property on="Dip for Protein" class="Bool (strict)"("Val(Sgnl)"=TRUE ("Value (Signaling)")) -> ()  [unwired: 2 in, 2 out]
                    n592 = local write "Scripts"(T1."Dipping" ("Scripts")) -> ()
                  }
                }
              }
            }
          }
        }
      }
      event "Fixed Traps Data\nScript": Value Change {
        n593 = event-data() -> ()  [unwired: 1 in, 5 out]
        n594 = flat-sequence {
          frame #0 {
            n595 = case shown="True" "Green ON" {
              frame False {
              }
              frame True {
                n596 = property on="Green Laser ON" class="Bool (strict)"("Val(Sgnl)"=TRUE) -> ()  [unwired: 2 in, 2 out]
              }
            }
            n597 = local write "Offset (nm)"(0.0 ("Offset (nm)")) -> ()
            n598 = property on="Sample Channel\nFlow" class="Bool (strict)"("Val(Sgnl)"=FALSE ("Value (Signaling)")) -> ()  [unwired: 2 in, 2 out]
            n599 = property on="Trap Delta (MHz)" class="DigNum (strict)"("Val(Sgnl)"="Fixed Traps Trap Delta (MHz)") -> ()  [unwired: 2 in, 2 out]
          }
          frame #1 {
            n600 = Wait (ms)(milliseconds to wait=u32 1000) -> ()  [unwired: 1 out]
          }
          frame #2 {
            n601 = local write "Start Saving"(TRUE ("Start Saving")) -> ()
          }
          frame #3 {
            n602 = local read "Bead Sep. Int. Time (s)"() -> (w959:dbl)
            n603 = Multiply(x=w959, y=1000.0) -> (x*y=w961:dbl)
            n604 = Wait (ms)(milliseconds to wait=w961) -> ()  [unwired: 1 out]
          }
          frame #4 {
            n605 = property on="Remove Offset" class="Bool (strict)"("Val(Sgnl)"=TRUE ("Value (Signaling)")) -> ()  [unwired: 2 in, 2 out]
          }
          frame #5 {
            n606 = property on="Dip for Protein" class="Bool (strict)"("Val(Sgnl)"="Start dipping after?") -> ()  [unwired: 2 in, 2 out]
          }
        }
      }
      event "Got DNA bead": Value Change {
        n607 = event-data() -> ()  [unwired: 1 in, 5 out]
        n608 = flat-sequence {
          frame #0 {
            n609 = local read "Daq spot flow on"() -> (w966:bool)
            n610 = case shown="True" w966 {
              frame False {
              }
              frame True {
                n611 = property on="Sample Channel\nFlow" class="Bool (strict)"("Val(Sgnl)"=TRUE ("Value (Signaling)")) -> ()  [unwired: 2 in, 2 out]
              }
            }
            n612 = property on="Got DNA bead" class="Bool"("Key Focus"=FALSE) -> ()  [unwired: 2 in, 2 out]
          }
          frame #1 {
            n613 = property on="Inject Pump 1" class="Bool (strict)"("Val(Sgnl)"=FALSE ("Value (Signaling)")) -> ()  [unwired: 2 in, 2 out]
          }
          frame #2 {
            n614 = property on="Cal/Data Acq. Spot" class="Bool (strict)"("Val(Sgnl)"=TRUE ("Value (Signaling)")) -> ()  [unwired: 2 in, 2 out]
          }
        }
      }
      event "Take Stepping Data": Value Change {
        n615 = event-data() -> ()  [unwired: 1 in, 5 out]
        n616 = local read "Save ave N"() -> (w978:dbl)
        n617 = flat-sequence {
          tunnel: w978 -> [w980]
          tunnel: [w980] -> w973
          tunnel: [w982] -> w974
          tunnel: w973 -> [w982]
          tunnel: [w984] -> w975
          tunnel: w974 -> [w984]
          tunnel: [w987] -> w976
          tunnel: w975 -> [w987]
          tunnel: [w989] -> w977
          tunnel: w976 -> [w989]
          tunnel: [w991] -> w971
          tunnel: w977 -> [w991]
          tunnel: w971 -> [w994]
          tunnel: [w994] -> w970
          tunnel: w970 -> [w995]
          tunnel: [w995] -> w972
          tunnel: w972 -> [w1001]
          frame #0 {
            n618 = property on="Save ave N" class="DigNum (strict)"("Val(Sgnl)"="Save ave factor") -> ()  [unwired: 2 in, 2 out]
          }
          frame #1 {
            n619 = Wait (ms)(milliseconds to wait=u32 100) -> ()  [unwired: 1 out]
          }
          frame #2 {
            n620 = local read "Offset 2 Start (MHz)"() -> (w986:dbl)
            n621 = property on="Saved AOD Raster Scan Parameter Sets" class="Arr (strict)"("Index Values"=u32[] [2]) -> ()  [unwired: 2 in, 2 out]
            n622 = property on="Trap Delta (MHz)" class="DigNum (strict)"("Val(Sgnl)"=w986) -> ()  [unwired: 2 in, 2 out]
          }
          frame #3 {
            n623 = property on="Load parameters" class="Bool (strict)"("Val(Sgnl)"=TRUE ("Value (Signaling)")) -> ()  [unwired: 2 in, 2 out]
          }
          frame #4 {
            n624 = Wait (ms)(milliseconds to wait=u32 100) -> ()  [unwired: 1 out]
          }
          frame #5 {
            n625 = property on="Trap Raster Scan" class="Bool (strict)"("Val(Sgnl)"=TRUE ("Value (Signaling)")) -> ()  [unwired: 2 in, 2 out]
          }
          frame #6 {
            n626 = Wait (ms)(milliseconds to wait=u32 1000) -> ()  [unwired: 1 out]
          }
          frame #7 {
            n627 = while {
              stop <- w998 stop-if-true
              n628 = local read "Raster Scanning..."() -> (w1000:bool)
              n629 = local read "Saving..."() -> (w999:bool)
              n630 = Not(x=w999) -> (.not. x?=w996:bool)
              n631 = Not(x=w1000) -> (.not. x?=w997:bool)
              n632 = And(x=w997, y=w996) -> (x .and. y?=w998:bool)
            }
          }
          frame #8 {
            n633 = property on="Save ave N" class="DigNum (strict)"("Val(Sgnl)"=w1001) -> ()  [unwired: 2 in, 2 out]
          }
        }
      }
      event "Step Size (nm)": Value Change {
        n634 = event-data() -> ()  [unwired: 1 in, 5 out]
        n635 = flat-sequence {
